vi "Multiply with Twiddle Factor.vi"(0 "Real{Input}":fxp<+/-,22,1>, 5 "Imag{Input}":fxp<+/-,22,1>, 7 "Real{Twiddle}":fxp<+/-,18,2>, 9 "Imag{Twiddle}":fxp<+/-,18,2>, 11 "Input Valid":bool) -> (4 "Real{Output}":fxp<+/-,19,2> format="%.18g", 6 "Imag{Output}":fxp<+/-,19,2> format="%.18g", 15 "Output Valid":bool)   [LabVIEW 2011]
doc: "This VI multiplies input data with twiddle factors\n\n<b> Scaling Down = 2 </b>\n<b>Latency = 6Ticks </b>"
uses:
  <vilib>/rvi/FXPMathLib/SharedSubVIs/typedef/nifxpmath_BASIC_ImplementationSettings.ctl
  <vilib>/fxp/LVFixedPointQuantizationPolicyTypeDef.ctl
  <vilib>/fxp/LVFixedPointOverflowPolicyTypeDef.ctl
  <vilib>/rvi/ClientSDK/Core/DevComputerLib/Private/FourWireProtocol(cint64).vi
  <vilib>/rvi/FXPMathLib/basic elements/FxpDiscreteDelay/XNode/nifxpmath_DiscreteDelay.xnode
  <vilib>/rvi/FXPMathLib/FxpMultComplex/XNode/niFpgaMultComplex.xnode
  <vilib>/rvi/XilinxIP/XIPIN_XNode/niFpgaXIPIN.xnode
  <vilib>/rvi/IPIntegrationNode/IPINode_Xnode/niFpgaIPINode.xnode
  <vilib>/rvi/IPIntegrationNode/IPINode_Utilities/niFpgaIPINodeSimCore.vi
  <userlib>/FPGA Library/Code Development/Signal Processing/FFT/Complex Multiply/Multiply with Twiddle Factor/Complex Multiplier/Complex_Multiplier_16754AB44A05940DE57C4E8178407981.dll
  <vilib>/rvi/ClientSDK/Core/DevComputerLib/niFpgaDevCompUtilities.lvlib
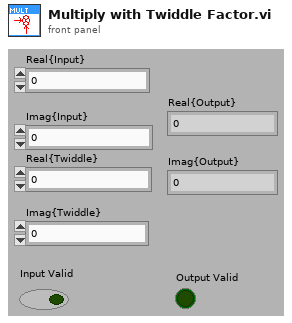
[diagram p1: front panel]
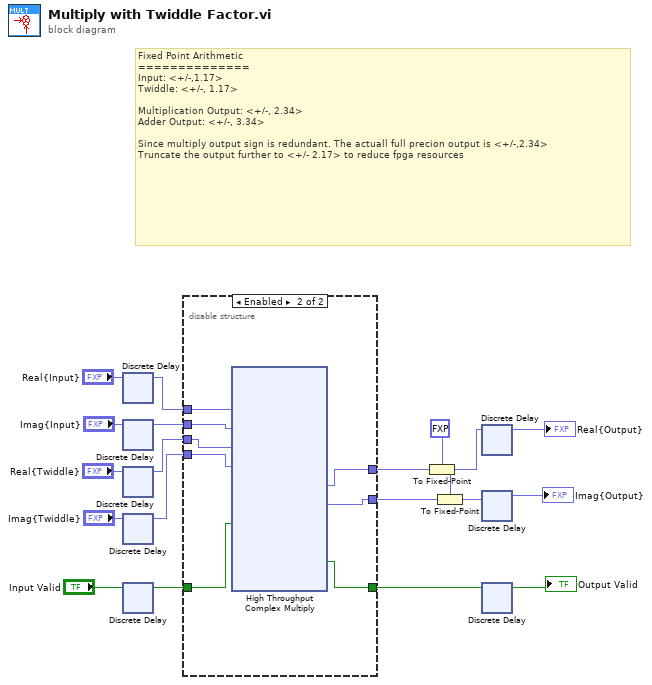
[diagram p0: block diagram]
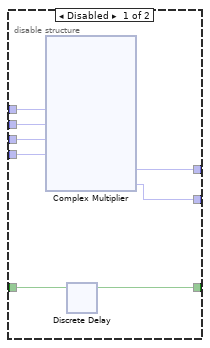
[diagram p2: hidden frame]
diagram:
  # "Fixed Point Arithmetic\n==============\nInput: <+/-,1.17>\nTwiddle: <+/-, 1.17>\n\nMultiplication Output: <+/-, 2.34>\nAdder Output: <+/-, 3.34>\n\nSince multiply output sign is redundant. The actuall full precion output is <+/-,2.34>\nTruncate the output further to <+/- 2.17> to reduce fpga resources"
  n1 = xnode "Discrete Delay"("D"="Real{Input}") -> ("Q"=w7:fxp<+/-,22,1>)
  n2 = xnode "Discrete Delay"("D"="Imag{Input}") -> ("Q"=w6:fxp<+/-,22,1>)
  n3 = xnode "Discrete Delay"("D"="Real{Twiddle}") -> ("Q"=w5:fxp<+/-,18,2>)
  n4 = xnode "Discrete Delay"("D"="Imag{Twiddle}") -> ("Q"=w4:fxp<+/-,18,2>)
  n5 = xnode "Discrete Delay"("D"="Input Valid") -> ("Q"=w3:bool)
  n6 = disable-structure shown="Enabled" {
    disable-tunnel: [w27 w79] -> w15
    disable-tunnel: [w26 w82] -> w14
    disable-tunnel: [w25 w81] -> w13
    disable-tunnel: w7 -> [w24 w86]
    disable-tunnel: w6 -> [w23 w85]
    disable-tunnel: w5 -> [w22 w84]
    disable-tunnel: w4 -> [w21 w83]
    disable-tunnel: w3 -> [w20 w80]
    frame Disabled {
      n7 = xnode ("Complex Multiplier")("ar"=w24, "ai"=w23, "br"=w22, "bi"=w21) -> ("pr"=w26:fxp<+/-,37,3>, "pi"=w25:fxp<+/-,37,3>)
      n8 = xnode "Discrete Delay"("D"=w20) -> ("Q"=w27:bool)
    }
    frame Enabled {
      n9 = xnode "High Throughput Complex Multiply"("xr"=w86, "xi"=w85, "yr"=w84, "yi"=w83, "input valid"=w80) -> ("pr"=w82:fxp<+/-,41,4>, "pi"=w81:fxp<+/-,41,4>, "output valid"=w79:bool)  [unwired: 1 in, 1 out]
    }
  }
  n10 = To Fixed-Point(fixed-point type=fxp<+/-,19,2> 0.0, number=w14) -> (fixed-point=w1:fxp<+/-,19,2>)
  n11 = To Fixed-Point(fixed-point type=w1, number=w13) -> (fixed-point=w12:fxp<+/-,19,2>)
  n12 = xnode "Discrete Delay"("D"=w1) -> ("Q"=→"Real{Output}":fxp<+/-,19,2>)
  n13 = xnode "Discrete Delay"("D"=w12) -> ("Q"=→"Imag{Output}":fxp<+/-,19,2>)
  n14 = xnode "Discrete Delay"("D"=w15) -> ("Q"=→"Output Valid":bool)
